vi "Add Chassis_Add Chassis.vi"(8 "error in (no error)":errorcluster, 10 "Settings":T1, 11 "Hardware Ref":refnum<k24>) -> (0 "error out":errorcluster, 3 "Hardware Ref Out":refnum<k24>)   [LabVIEW 2019, in "Simple SysDef API.lvlib"]
uses:
  <userlib>/SimpleSysDef/Simple SysDef API.lvlib
  NationalInstruments.VeriStand.SystemDefinitionAPI
  <userlib>/SimpleSysDef/_SubVIs/Add Chassis_Settings.ctl
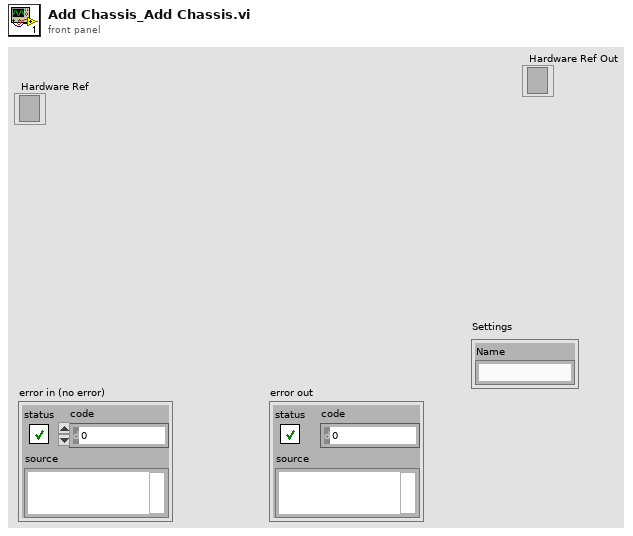
[diagram p1: front panel]
types:
  T1 = typedef "Simple SysDef API.lvlib/Add Chassis_Settings.ctl" = cluster{"Name":string}
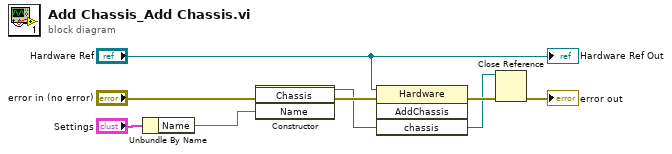
[diagram p0: block diagram]
diagram:
  n1 = Unbundle By Name("Settings") -> ("Name"=w7:string)
  n2 = constructor class="Chassis"(error in="error in (no error)", "Name"=w7) -> (reference out=w1:refnum<k24>, error out=w2:errorcluster)  [unwired: 2 in, 2 out]
  n3 = invoke class="Hardware" method="AddChassis"(reference="Hardware Ref", error in=w2, "chassis"=w1) -> (error out=w6:errorcluster)  [unwired: 1 in, 3 out]
  n4 = Close Reference(reference=w1, error in (no error)=w6) -> (error out=→"error out":errorcluster)
  "Hardware Ref Out" <- "Hardware Ref"
